vi "get parameters.vi"(8 "error in (no error)":errorcluster caption="Fehler (Eingang, kein Fehler)", 11 "TestInterface (Eingang)":refnum<class "TestInterface.lvclass">) -> (0 "error out":errorcluster caption="Fehler (Ausgang)", 2 "parameters":string[](array[string]), 3 "TestInterface (Ausgang)":refnum<class "TestInterface.lvclass">)   [LabVIEW 2013, in "TestInterface.lvclass"]
uses:
  TestInterface.lvclass
  TestInterface.lvclass/TestInterface.ctl
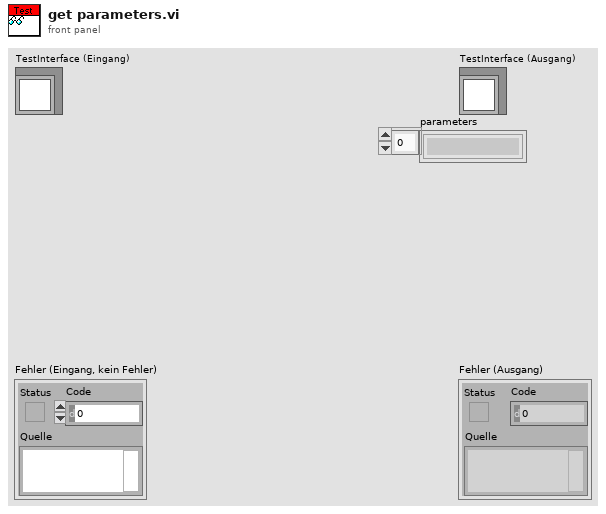
[diagram p1: front panel]
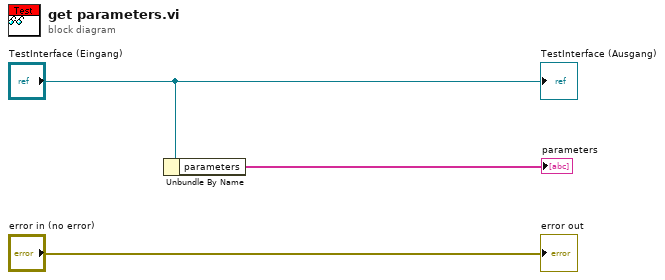
[diagram p0: block diagram]
diagram:
  n1 = Unbundle By Name("TestInterface (Eingang)") -> ("parameters"=→"parameters":string[])
  "error out" <- "error in (no error)"
  "TestInterface (Ausgang)" <- "TestInterface (Eingang)"
